vi "Regler FT-IR HP.vi"(7 "Index":i32, 8 "Fehler":errorcluster caption="Fehler (Eingang)") -> (0 "Fehler (Ausgang)":errorcluster)   [LabVIEW 2020, in "Regler.lvlib" / "Druckregler.lvlib"]
uses:
  Druckregler.lvlib
  Aktionen Param. Druckregler.ctl
  Aktionen Interne Werte.ctl
  Verwaltung/FGV IN Aktionen.ctl
  Konfig-Dateien/FGV Betriebsdaten Aktionen.ctl
  Verwaltung/FGV OUT Aktionen.ctl
  Allgemein/Aktionen FGV Dichtheitstest.ctl
  Allgemein/FGV Zustaende Aktionen.ctl
  Funktionstasten/Zustaende.ctl
  Visualisierungs Elemente/Zahlen-Eingabefeld.ctl
  Verwaltung/Verwaltung - cRIO.lvlib
  Allgemein/Allgemein.lvlib
  Konfig-Dateien/Konfig-Dateien.lvlib
  Funktionstasten/Funktionstasten.lvlib
  Regler.lvlib
  Aktion FGV Werte vorgeben.ctl
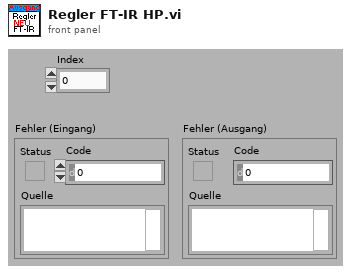
[diagram p1: front panel]
types:
  T1 = typedef "Zahlen-Eingabefeld.ctl" = sgl
  T2 = typedef "Funktionstasten.lvlib/Zustaende.ctl" = enum16{"Standby", "Pause", "Eco", "Messen", "Kalibrieren", "Spülen Filter", "Spülen Leitung", "Umgebungsluft", "0-Gas", "Cal-Gas", "CG zu PNS", "-------------", "Init 1", "Init 2", "Init 3", "Init 4", "Messen vorbereiten", "Messen durchführen", "Exit"}
  T3 = typedef "Allgemein.lvlib/FGV Zustaende Aktionen.ctl" = enum16{"lesen", "Zustand PC", "Zustand cRIO", "Bildnummer", "Samplepoint", "Sysloglevel"}
  T4 = typedef "Allgemein.lvlib/Aktionen FGV Dichtheitstest.ctl" = enum16{"lesen", "schreiben"}
  T5 = typedef "Verwaltung - cRIO.lvlib/FGV OUT Aktionen.ctl" = enum16{"lesen", "ANA OUT", "DO 0-31", "DO 32-47"}
  T6 = typedef "Konfig-Dateien.lvlib/FGV Betriebsdaten Aktionen.ctl" = enum16{"lesen", "Anlagengrenzw.", "PID Param.", "Sonstige", "Sensor Para."}
  T7 = typedef "Verwaltung - cRIO.lvlib/FGV IN Aktionen.ctl" = enum16{"lesen", "DI", "AI", "Fühler Br.", "TC", "Fühler Br. TC"}
  T8 = typedef "Regler.lvlib/Druckregler.lvlib/Aktionen Interne Werte.ctl" = enum16{"lesen", "FT-IR", "Ausgang", "Pumpe", "laden", "speichern", "Änderung?", "Druck Kalter Block", "Dichtheitstest"}
  T9 = typedef "Regler.lvlib/Druckregler.lvlib/Aktionen Param. Druckregler.ctl" = enum16{"lesen", "schreiben", "Regler FT-IR", "Regler Ausgang", "Regler Durchfluss", "Regler PMA", "Regler NDIR", "Regler Filterblock", "Regler Gaskühler", "Regler Kalter Block"}
  T10 = typedef "Anlagengrenzwerte.lvlib/Anlagen-Grenzwerte Anzeige.ctl" = cluster{"Eingangsdruck FT-IR:":T11, "Durchfluss FT-IR:":T11, "Durchfluss CalGas:":T11, "Druck Ausgang:":T11, "Druck Kalter Block:":T11, "Heizleitungen intern:":T11, "Heizleitung zu FT-IR:":T11, "Heizung Filterblock:":T11, "Heizung Pumpe:":T11, "Heizleitung Extern SP1:":T11, "Heizleitung Extern SP2:":T11, "FT-IR Heizung Messzelle:":T11, "Schaltschranktemperatur:":T11, "Gaskühler:":T11}
  T11 = typedef "Anlagengrenzwerte.lvlib/Anlagen-Parameter Anzeige.ctl" = cluster{"Sollwert":sgl, "Warn-Min":sgl, "Warn-Max":sgl, "Abschalt-Min":sgl, "Abschalt-Max":sgl, "Regler":u16}
  T12 = typedef "Verwaltung - cRIO.lvlib/Analog Eingaenge.ctl" = cluster{"AI0: Durchfluss FT-IR":sgl, "AI1: Druck Ausgang":sgl, "AI2: Umgebungsdruck":sgl, "AI3: Druck FT-IR":sgl, "AI4: Druck CalGas":sgl, "AI5: Reserve":sgl, "AI6: Reserve":sgl, "AI7: Reserve":sgl, "Rohwert Durchfluss FT-IR":sgl, "Rohwert Druck Ausgang":sgl, "Rohwert Umgebungsdruck":sgl, "Rohwert Druck FT-IR":sgl, "Rohwert Druck CalGas":sgl, "Rohwert AI5":sgl, "Rohwert AI6":sgl, "Rohwert AI7":sgl, "Rohwert Diffdruck mbar FTIR":sgl}
  T13 = typedef "Verwaltung - cRIO.lvlib/Digital Ausgaenge 0-31.ctl" = cluster{"O0: Druckluft Versorgung":bool, "O1: CG 1 (FB Eingang 1)":bool, "O2: CG 2 (Kühlung FT-IR EIN)":bool, "O3: CG 3 (FB Bypass)":bool, "O4: CG 4 (FB CalGas)":bool, "O5: CG 5 (FB spülen/UL)":bool, "O6: CG 6 (FB zum FT-IR)":bool, "O7: CG 7 (FB zum FID)":bool, "O8: CG 8 (FB Reserve)":bool, "O9: (FB Reserve)":bool, "O10: (FB Umgebungsluft FID)":bool, "O11: (FB zum Gaskühler)":bool, "O12: FB Stickstoff zu FT-IR":bool, "O13: Optikbox FT-IR spülen":bool, "O14: (Purifier deaktivieren)":bool, "O15: (Umschaltung Purifier/Stickstoff)":bool, "O16: N2 Einblasung":bool, "O17: LSP LN2 Nachfüllung":bool, "O18: (Reserve)":bool, "O19: (Pumpe Eingang1)":bool, "O20: (Pumpe Eingang2)":bool, "O21: (Pumpe Spülen1)":bool, "O22: (Pumpe Spülen2)":bool, "O23: (Reserve)":bool, "O24: CalGas 1":bool, "O25: CalGas 2":bool, "O26: CG 3-8 (CalGas 3)":bool, "O27: Stickstoff aufschalten":bool, "O28: CG zu PNS":bool, "O29: FTIR Standby Spülung":bool, "O30: CG zu Entnahme(T90)":bool, "O31: (Purifier regenerieren)":bool}
  T14 = typedef "Verwaltung - cRIO.lvlib/Analog Eingaenge.ctl" = cluster{"AI0: Durchfluss FT-IR":sgl, "AI1: Druck Ausgang":sgl, "AI2: Umgebungsdruck":sgl, "AI3: Druck FT-IR":sgl, "AI4: Druck CalGas":sgl, "AI5: Taupunktsensor":sgl, "AI6: Reserve":sgl, "AI7: Druck CG PMA":sgl, "AI8: Durchfluss PMA":sgl, "AI9: Druck Kalter Block":sgl, "AI10: Umgebungsdruck(reserve)":sgl, "AI11: Temperatur Gaskühler":sgl, "AI12: Reserve":sgl, "AI13: Reserve":sgl, "AI14: Reserve":sgl, "AI15: Reserve":sgl, "Rohwert Durchfluss FT-IR":sgl, "Rohwert Druck Ausgang":sgl, "Rohwert Umgebungsdruck":sgl, "Rohwert Druck FT-IR":sgl, "Rohwert AI4":sgl, "Rohwert AI5":sgl, "Rohwert AI6":sgl, "Rohwert AI7":sgl, "Rohwert AI8":sgl, "Rohwert AI9":sgl, "Rohwert AI10":sgl, "Rohwert AI11":sgl, "Rohwert AI12":sgl, "Rohwert AI13":sgl, "Rohwert AI14":sgl, "Rohwert AI15":sgl, "Rohwert Diffdruck mbar FTIR":sgl}
  T15 = cluster{"Numerisch":sgl, "Numerisch":sgl, "Numerisch":sgl, "Numerisch":sgl, "Numerisch":sgl}
  T16 = typedef "Regler.lvlib/Druckregler.lvlib/Regler Interne Werte.ctl" = cluster{"PV":sgl, "D-action":sgl, "Error":sgl, "I-action":sgl, "OUT":sgl}
  T17 = typedef "Erweiterte Konfig.lvlib/Aktionen Dichtheitstest.ctl" = enum16{"Initialisieren", "Unterdruck aufbauen", "Prop schließen", "Warten", "Auswertung", "Fertig"}
  T18 = typedef "Regler.lvlib/Aktion FGV Werte vorgeben.ctl" = enum16{"lesen", "P-Flow", "D-Filterblock"}
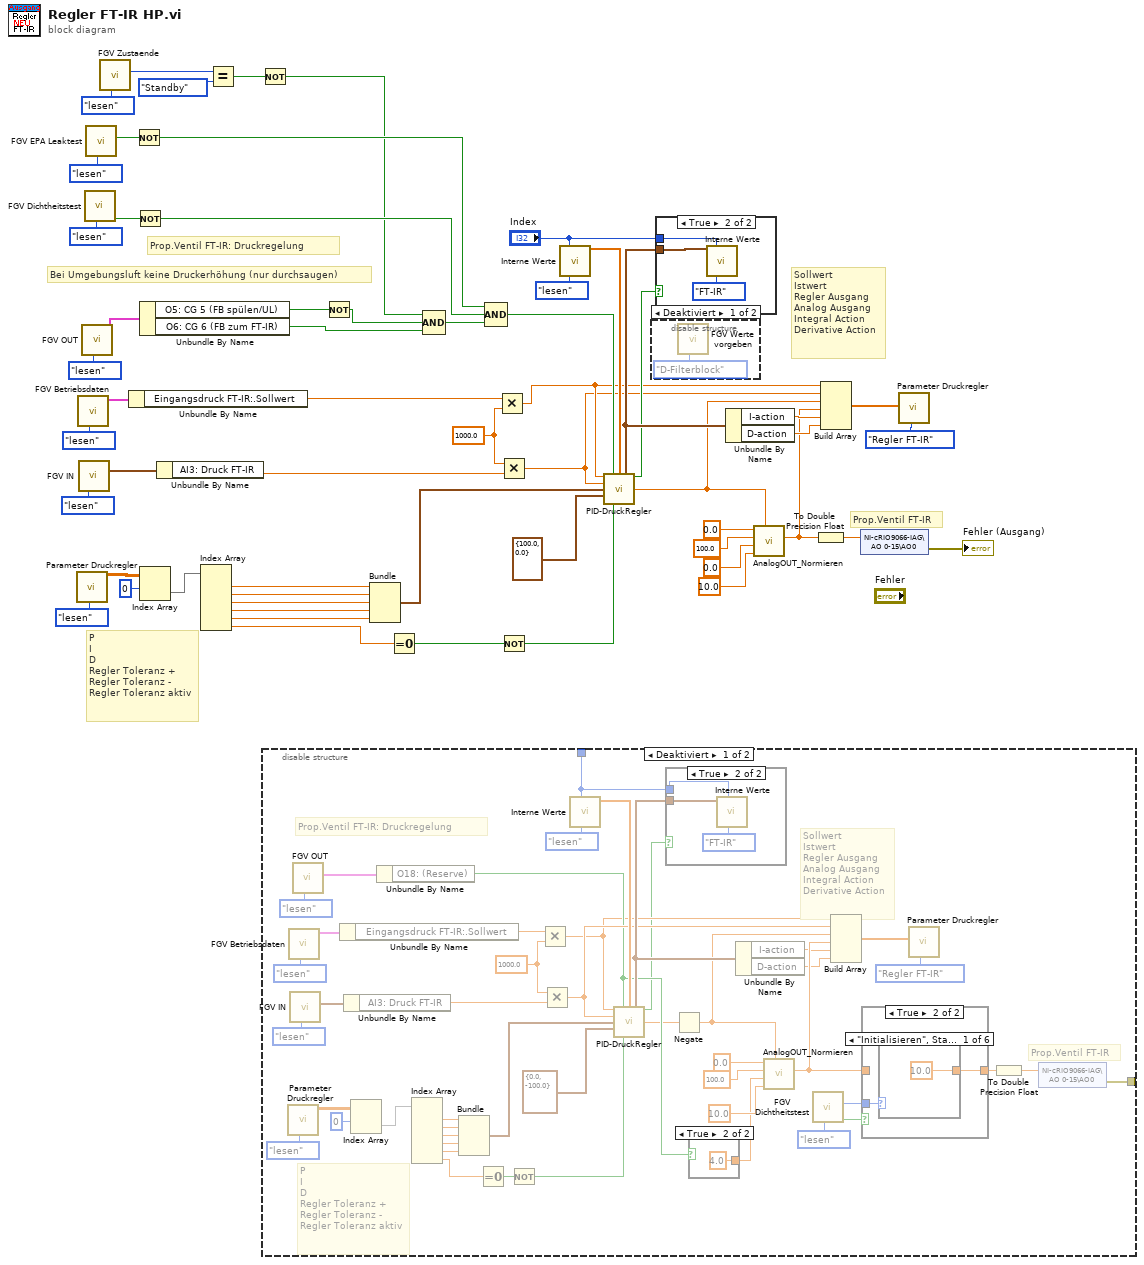
[diagram p0: block diagram]
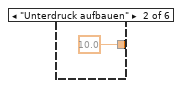
[diagram p6: hidden frame]
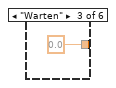
[diagram p7: hidden frame]
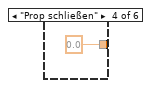
[diagram p8: hidden frame]
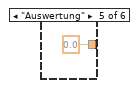
[diagram p9: hidden frame]
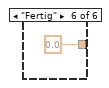
[diagram p10: hidden frame]
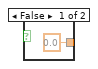
[diagram p11: hidden frame]
diagram:
  w5 = T1 1000.0 ("y")
  # "Bei Umgebungsluft keine Druckerhöhung (nur durchsaugen)"
  # "Prop.Ventil FT-IR"
  # "Prop.Ventil FT-IR: Druckregelung"
  # "Sollwert\nIstwert\nRegler Ausgang\nAnalog Ausgang\nIntegral Action\nDerivative Action"
  # "P\nI\nD\nRegler Toleranz +\nRegler Toleranz -\nRegler Toleranz aktiv"
  n1 = call "Parameter Druckregler.vi"("Aktionen"=Aktionen_Param._Druckregler."lesen") -> ("Regleparameter"=w39:sgl[][])  [unwired: 10 in, 8 out]
  n2 = call "FGV Betriebsdaten.vi"("Aktionen"=FGV_Betriebsdaten_Aktionen."lesen") -> ("Anlagen-Grenzwerte"=w25:T10)  [unwired: 7 in, 3 out]
  n3 = call "FGV IN.vi"("Aktion"=FGV_IN_Aktionen."lesen") -> ("Analog Eingänge"=w24:T12)  [unwired: 10 in, 4 out]
  n4 = call "FGV OUT.vi"("Aktion"=FGV_OUT_Aktionen."lesen") -> ("DO 0-31"=w26:T13)  [unwired: 7 in, 3 out]
  n5 = call "FGV Dichtheitstest.vi"("Aktionen"=Aktionen_FGV_Dichtheitstest."lesen") -> ("Dichtheitstest?"=w21:bool)  [unwired: 9 in, 1 out]
  n6 = call "FGV EPA Leaktest.vi"("Aktion"=enum16{"lesen", "schreiben"}."lesen") -> ("Leaktest aktiv"=w14:bool)  [unwired: 9 in, 1 out]
  n7 = call "FGV Zustaende.vi"("Aktionen"=FGV_Zustaende_Aktionen."lesen") -> ("Zustand cRIO"=w7:T2)  [unwired: 6 in, 4 out]
  n8 = Unbundle By Name(w25) -> ("Eingangsdruck FT-IR:.Sollwert"=w4:sgl)
  n9 = Not(x=w14) -> (.not. x?=w13:bool)
  n10 = Not(x=w21) -> (.not. x?=w20:bool)
  n11 = Unbundle By Name(w26) -> ("O5: CG 5 (FB spülen/UL)"=w17:bool, "O6: CG 6 (FB zum FT-IR)"=w18:bool)
  n12 = Index Array(array=w39, index (row)=0 ("Deaktivierter Index (Spalte)")) -> (element=w38:sgl[])  [unwired: 1 in]
  n13 = Unbundle By Name(w24) -> ("AI3: Druck FT-IR"=w1:sgl)
  n14 = Index Array(array=w38) -> (element #1=w50:sgl, element #2=w49:sgl, element #3=w48:sgl, element #4=w47:sgl, element #5=w46:sgl, element #6=w34:sgl)  [unwired: 6 in]
  n15 = Equal?(x=w7, y=Zustaende."Standby") -> (x = y?=w8:bool)
  n16 = Not(x=w8) -> (.not. x?=w9:bool)
  n17 = disable-structure shown="Deaktiviert" {
    disable-tunnel: _ -> [w69 _]
    disable-tunnel: [w65 _] -> _
    frame Disabled {
      w84 = T1 1000.0 ("y")
      # "Prop.Ventil FT-IR"
      # "Prop.Ventil FT-IR: Druckregelung"
      # "Sollwert\nIstwert\nRegler Ausgang\nAnalog Ausgang\nIntegral Action\nDerivative Action"
      # "P\nI\nD\nRegler Toleranz +\nRegler Toleranz -\nRegler Toleranz aktiv"
      n18 = call "Parameter Druckregler.vi"("Aktionen"=Aktionen_Param._Druckregler."lesen") -> ("Regleparameter"=w89:sgl[][])  [unwired: 7 in, 3 out]
      n19 = call "FGV Betriebsdaten.vi"("Aktionen"=FGV_Betriebsdaten_Aktionen."lesen") -> ("Anlagen-Grenzwerte"=w60:T10)  [unwired: 7 in, 3 out]
      n20 = call "FGV IN.vi"("Aktion"=FGV_IN_Aktionen."lesen") -> ("Analog Eingänge"=w59:T14)  [unwired: 8 in, 2 out]
      n21 = call "FGV OUT.vi"("Aktion"=FGV_OUT_Aktionen."lesen") -> ("DO 0-31"=w61:T13)  [unwired: 7 in, 3 out]
      n22 = Unbundle By Name(w60) -> ("Eingangsdruck FT-IR:.Sollwert"=w85:sgl)
      n23 = Unbundle By Name(w59) -> ("AI3: Druck FT-IR"=w83:sgl)
      n24 = Index Array(array=w89, index (row)=0 ("Deaktivierter Index (Spalte)")) -> (element=w88:sgl[])  [unwired: 1 in]
      n25 = Unbundle By Name(w61) -> ("O18: (Reserve)"=w74:bool)
      n26 = Index Array(array=w88) -> (element #1=w100:sgl, element #2=w99:sgl, element #3=w98:sgl, element #4=w97:sgl, element #5=w96:sgl, element #6=w71:sgl)  [unwired: 6 in]
      n27 = Bundle("Numerisch"=w100, "Numerisch"=w99, "Numerisch"=w98, "Numerisch"=w97, "Numerisch"=w96) -> (w94:T15)  [unwired: 1 in]
      n28 = Equal To 0?(x=w71) -> (x = 0?=w95:bool)
      n29 = Not(x=w95) -> (.not. x?=w93:bool)
      n30 = Multiply(x=w85, y=w84) -> (x*y=w73:T1)
      n31 = Multiply(x=w84, y=w83) -> (x*y=w82:T1)
      n32 = call "Interne Werte.vi"("Aktionen Interne Werte"=Aktionen_Interne_Werte."lesen", "Index"=w69) -> ("FT-IR"=w106:sgl[])  [unwired: 4 in, 5 out]
      n33 = call "PID-DruckRegler.vi"("Sollwert"=w73, "Regler EIN"=w74, "Regler Interne Werte"=w106, "Istwert"=w82, "PID-Parameter"=w94, "output range"=cluster{"output high":dbl, "output low":dbl} {"output high"=0.0, "output low"=-100.0}, "Regler Toleranz verwenden?"=w93) -> ("Regler Interne Werte"=w105:T16, "Interne Werte speichern"=w68:bool, "Output"=w72:sgl)  [unwired: 6 in]
      n34 = case shown="True" w68 {
        tunnel: w69 -> [_ w108]
        tunnel: w105 -> [_ w107]
        frame False {
        }
        frame True {
          n35 = call "Interne Werte.vi"("Aktionen Interne Werte"=Aktionen_Interne_Werte."FT-IR", "Index"=w108, "Regler Interne Werte"=w107) -> ()  [unwired: 3 in, 6 out]
        }
      }
      n36 = Negate(x=w72) -> (-x=w75:sgl)
      n37 = case shown="True" w74 {
        tunnel: [sgl 0.0 ("Untergrenze") sgl 4.0 ("Untergrenze")] -> w92
        frame False {
        }
        frame True {
        }
      }
      n38 = Unbundle By Name(w105) -> ("I-action"=w67:sgl, "D-action"=w66:sgl)
      n39 = call "AnalogOUT_Normieren.vi"("Analogwert"=w75, "Obergrenze"=sgl 10.0, "Untergrenze"=w92, "Max Analogwert"=sgl 100.0, "Min Analogwert"=sgl 0.0) -> ("Normierter Wert"=w79:sgl)  [unwired: 6 in]
      n40 = call "FGV Dichtheitstest.vi"("Aktionen"=Aktionen_FGV_Dichtheitstest."lesen") -> ("Dichtheitstest?"=w76:bool, "Aktionen Dichtheitstest"=w77:T17)  [unwired: 9 in]
      n41 = Build Array(w73, w82, w75, w79, w67, w66) -> (w87:T1[])
      n42 = case shown="True" w76 {
        tunnel: w77 -> [_ w112]
        tunnel: w79 -> [w110 _]
        tunnel: [w110 w111] -> w78
        frame False {
        }
        frame True {
          n43 = case shown="\"Initialisieren\", Standard" w112 {
            tunnel: [sgl 10.0 ("Untergrenze") sgl 10.0 ("Untergrenze") sgl 0.0 ("Untergrenze") sgl 0.0 ("Untergrenze") sgl 0.0 ("Untergrenze") sgl 0.0 ("Untergrenze")] -> w111
            frame "Initialisieren", Default {
            }
            frame "Unterdruck aufbauen" {
            }
            frame "Warten" {
            }
            frame "Prop schließen" {
            }
            frame "Auswertung" {
            }
            frame "Fertig" {
            }
          }
        }
      }
      n44 = call "Parameter Druckregler.vi"("Aktionen"=Aktionen_Param._Druckregler."Regler FT-IR", "Werte FT-IR"=w87) -> ()  [unwired: 6 in, 4 out]
      n45 = To Double Precision Float(number=w78) -> (double precision float=w81:dbl)
      n46 = shared-variable "NI-cRIO9066-IAG\\AO 0-15\\AO0"(w81) -> (error out=w65:errorcluster)  [unwired: 1 in]
    }
    frame Enabled {
    }
  }
  n47 = Not(x=w17) -> (.not. x?=w16:bool)
  n48 = Bundle("Numerisch"=w50, "Numerisch"=w49, "Numerisch"=w48, "Numerisch"=w47, "Numerisch"=w46) -> (w44:T15)  [unwired: 1 in]
  n49 = Equal To 0?(x=w34) -> (x = 0?=w45:bool)
  n50 = Compound Arithmetic op=AND ("Mehrfacharithmetik")(w9, w16, w18) -> (w19:bool)
  n51 = Compound Arithmetic op=AND ("Mehrfacharithmetik")(w13, w20, w19) -> (w10:bool)
  n52 = Multiply(x=w4, y=w5) -> (x*y=w3:T1)
  n53 = Multiply(x=w5, y=w1) -> (x*y=w2:T1)
  n54 = Not(x=w45) -> (.not. x?=w43:bool)
  n55 = call "Interne Werte.vi"("Index"="Index", "Aktionen Interne Werte"=Aktionen_Interne_Werte."lesen") -> ("FT-IR"=w56:sgl[])  [unwired: 7 in, 6 out]
  n56 = call "PID-DruckRegler.vi"("Sollwert"=w3, "Regler EIN"=w10, "Regler Interne Werte"=w56, "Istwert"=w2, "PID-Parameter"=w44, "output range"=cluster{"output high":dbl, "output low":dbl} {"output high"=100.0, "output low"=0.0}, "Regler Toleranz verwenden?"=w43) -> ("Regler Interne Werte"=w55:T16, "Interne Werte speichern"=w32:bool, "Output"=w6:sgl)  [unwired: 6 in]
  n57 = disable-structure shown="Deaktiviert" {
    frame Disabled {
      n58 = call "FGV Werte vorgeben.vi"("Aktion"=Aktion_FGV_Werte_vorgeben."D-Filterblock") -> ()  [unwired: 9 in, 2 out]
    }
    frame Enabled {
    }
  }
  n59 = case shown="True" w32 {
    tunnel: "Index" -> [_ w123]
    tunnel: w55 -> [_ w122]
    frame False {
    }
    frame True {
      n60 = call "Interne Werte.vi"("Regler Interne Werte"=w122, "Index"=w123, "Aktionen Interne Werte"=Aktionen_Interne_Werte."FT-IR") -> ()  [unwired: 6 in, 7 out]
    }
  }
  n61 = Unbundle By Name(w55) -> ("I-action"=w31:sgl, "D-action"=w30:sgl)
  n62 = call "AnalogOUT_Normieren.vi"("Analogwert"=w6, "Obergrenze"=sgl 10.0, "Untergrenze"=sgl 0.0, "Max Analogwert"=sgl 100.0, "Min Analogwert"=sgl 0.0) -> ("Normierter Wert"=w23:sgl)  [unwired: 6 in]
  n63 = To Double Precision Float(number=w23) -> (double precision float=w35:dbl)
  n64 = Build Array(w3, w2, w6, w23, w31, w30) -> (w37:T1[])
  n65 = shared-variable "NI-cRIO9066-IAG\\AO 0-15\\AO0"(w35) -> (error out=→"Fehler (Ausgang)":errorcluster)  [unwired: 1 in]
  n66 = call "Parameter Druckregler.vi"("Werte FT-IR"=w37, "Aktionen"=Aktionen_Param._Druckregler."Regler FT-IR") -> ()  [unwired: 9 in, 9 out]
